vi "Clip Data Write.vi"(8 "error in (no error)":errorcluster, 9 "Clip Data?":bool, 11 "3D Plot.lvclass in":refnum<class "3D Plot.lvclass">) -> (0 "error out":errorcluster, 3 "3D Plot.lvclass out":refnum<class "3D Plot.lvclass">)   [LabVIEW 2020, in "3D Plot.lvclass"]
uses:
  <vilib>/Math Plots/3D Math Plots/3D Plot/3D Plot/3D Plot.lvclass
  <vilib>/Math Plots/3D Math Plots/3D Plot/3D Plot/3D Plot.lvclass/3D Plot.ctl
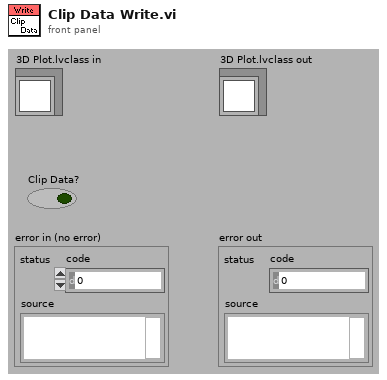
[diagram p1: front panel]
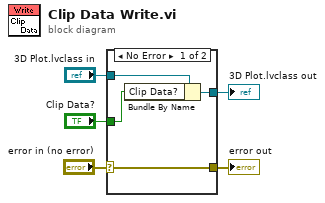
[diagram p0: block diagram]
diagram:
  n1 = case shown="No Error" "error in (no error)" {
    selector: "error in (no error)" -> [w6 w11]
    tunnel: "Clip Data?" -> [w9 _]
    tunnel: "3D Plot.lvclass in" -> [w8 w10]
    tunnel: [w7 w10] -> w3
    tunnel: [w6 w11] -> w1
    frame No Error {
      n2 = Bundle By Name(cluster=w8, "Clip Data?"=w9) -> (w7:refnum<class "3D Plot.lvclass">)
    }
    frame Error {
    }
  }
  "error out" <- w1
  "3D Plot.lvclass out" <- w3
